vi "Read DBL Pointer.vi"(8 "error in (no error)":errorcluster, 10 "buffer in":dbl[](array[numeric]), 11 "DBL Pointer in":refnum<class "DBL Pointer.lvclass">) -> (0 "error out":errorcluster, 2 "buffer out":dbl[](array[numeric]), 3 "DBL Pointer out":refnum<class "DBL Pointer.lvclass">)   [LabVIEW 2017, in "DSF Core.lvlib" / "DBL Pointer.lvclass"]
uses:
  DBL Pointer.lvclass
  C:/Program Files (x86)/National Instruments/LabVIEW 2017/vi.lib/NI/Memory Manager/Classes/Pointer/Memory.Pointer.lvclass
  DBL Pointer.lvclass/DBL Pointer.ctl
  <vilib>/NI/Memory Manager/Classes/Pointer/Memory.Pointer.lvclass/Memory.Pointer.ctl
  <vilib>/NI/Memory Manager/Classes/Pointer/Memory.Pointer.Read.1D.DBL.vi
  <vilib>/NI/Memory Manager/Classes/Pointer/Memory.Pointer.Read.No Check.1D.DBL.vi
  <vilib>/NI/Memory Manager/Classes/Pointer/Memory.Pointer.Parameter Check.Null Pointer.vi
  <vilib>/NI/Memory Manager/Classes/Pointer/Memory.Pointer.Parameter Check.Subset.Power of 2.vi
  <vilib>/NI/Memory Manager/Classes/Pointer/Memory.Pointer.Get Address.vi
  <vilib>/NI/Memory Manager/Classes/Pointer/Memory.Pointer.Errors.vi
  <vilib>/NI/Memory Manager/Classes/Pointer/Memory.Pointer.Errors.Null Pointer.vi
  <vilib>/NI/Memory Manager/Classes/Pointer/Memory.Pointer.Errors.Out of Bounds.vi
  <vilib>/NI/Memory Manager/Classes/Pointer/Memory.Pointer.Get Size.vi
  <vilib>/NI/Memory Manager/Classes/Pointer/Memory.Pointer.Count to Size.Power of 2.vi
  <vilib>/NI/Memory Manager/Classes/Pointer/Memory.Pointer.Errors.Create Error.vi
  <vilib>/NI/Memory Manager/VIs/Source.Write.String.vi
  <vilib>/NI/Memory Manager/Classes/Pointer/Memory.Pointer.Errors.Write Pointer Size.vi
  <vilib>/NI/Memory Manager/VIs/Source.Write.Scalar.Base10.vi
  <vilib>/NI/Memory Manager/VIs/Source.Write.Scalar.Base10 (U64).vi
  <vilib>/NI/Memory Manager/VIs/New Error Cluster Constant.vi
  <vilib>/NI/Memory Manager/VIs/New Error Cluster Constant (512B).vi
  <vilib>/NI/Memory Manager/VIs/Error Cluster.Set Status.vi
  <vilib>/NI/Memory Manager/VIs/Error Cluster.Set Code.vi
  <vilib>/NI/Memory Manager/VIs/Error Cluster.Set VI Source.vi
  <vilib>/NI/Memory Manager/Constants/Memory.Constants.vi
  <vilib>/NI/Memory Manager/Constants/Memory.Constants.Library Name.vi
  <vilib>/NI/Memory Manager/Classes/Pointer/Memory.Pointer.Errors.Get Info.vi
  <vilib>/NI/Memory Manager/Classes/Pointer/Memory.Pointer.lvclass
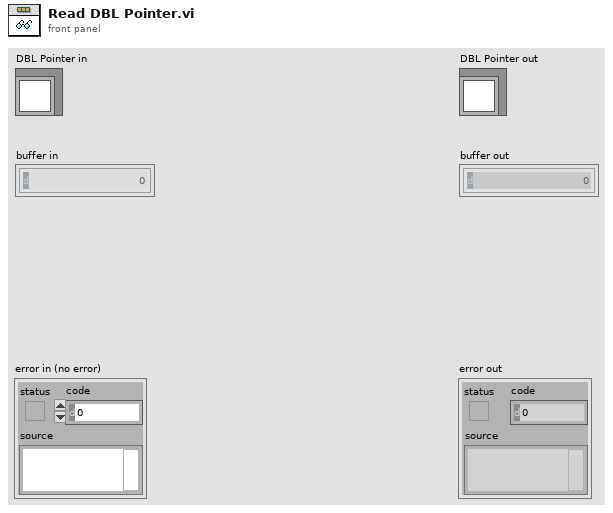
[diagram p1: front panel]
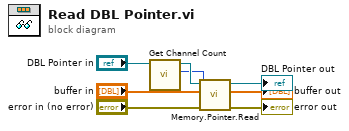
[diagram p0: block diagram]
diagram:
  n1 = call "Get Channel Count.vi"("DBL Buffer in"="DBL Pointer in") -> ("channel count"=w3:u64, "DBL Buffer out"=w4:refnum<class "DBL Pointer.lvclass">)  [unwired: 9 in]
  n2 = call-poly <vilib>:"Memory.Pointer.Read.vi"("error in (no error)"="error in (no error)", "offset (0)"=w3, "buffer in"="buffer in", "Pointer in"=w4) -> ("error out"=→"error out":errorcluster, "buffer out"=→"buffer out":dbl[], "Pointer out"=→"DBL Pointer out":refnum<class "DBL Pointer.lvclass">)  [unwired: 4 in, 1 out]
